vi "S7COMM - Parse Response - Decode Data Item.vi"(8 "error in (no error)":errorcluster, 9 "Variable Type":T1=enum."BIT", 11 "Response Data IN":T2 format="0x%02x") -> (0 "error out":errorcluster, 2 "Read Item - Data":i32[](array[numeric]), 3 "Response Data OUT":T2 format="0x%02x")   [LabVIEW 2014, in "S7NetCom.lvclass"]
doc: "____\nCopyright (c) 2019 Hampel Software Engineering (HSE), released under BSD license. More info can be found on https://dokuwiki.hampel-soft.com/code/hse/s7netcom. Original code published by Marc Christenson, Sisu Devices."
uses:
  S7NetCom.lvclass
  Controls/S7NetCom_HexByteArray.ctl
  Controls/S7NetCom_HexByte.ctl
  Controls/S7_Variable_Type.ctl
  S7COMM - Evaluate Response Item Return Code.vi
  S7COMM - Response Item Return Code-error.vi
panel:
  # "More info on https://dokuwiki.hampel-soft.com/code/hse/s7netcom\n\nCopyright (c) 2019, HAMPEL SOFTWARE ENGINEERING (HSE)\nOriginal code developed by Marc Christenson, Sisu Devices\nAll rights reserved.\n\nRedistribution and use in source and binary forms, with or without\nmodification, are permitted provided that the following conditions are met:\n\n1. Redistributions of source code must retain the above copyright\n   notice, this list of conditions and the following disclaimer.\n\n2. Redistributions in binary form must reproduce the above copyright\n   notice, this list of conditions and the following disclaimer in the\n   documentation and/or other materials provided with the distribution.\n\n3. All advertising materials mentioning features or use of this software\n   must display the following acknowledgement:\n   This product includes software developed by HAMPEL SOFTWARE ENGINEERING.\n\n4. Neither the name of HAMPEL SOFTWARE ENGINEERING nor the\n   names of its contributors may be used to endorse or promote products\n   derived from this software without specific prior written permission.\n\nTHIS SOFTWARE IS PROVIDED BY HAMPEL SOFTWARE ENGINEERING ''AS IS'' AND ANY\nEXPRESS OR IMPLIED WARRANTIES, INCLUDING, BUT NOT LIMITED TO, THE IMPLIED\nWARRANTIES OF MERCHANTABILITY AND FITNESS FOR A PARTICULAR PURPOSE ARE\nDISCLAIMED. IN NO EVENT SHALL HAMPEL SOFTWARE ENGINEERING BE LIABLE FOR ANY\nDIRECT, INDIRECT, INCIDENTAL, SPECIAL, EXEMPLARY, OR CONSEQUENTIAL DAMAGES\n(INCLUDING, BUT NOT LIMITED TO, PROCUREMENT OF SUBSTITUTE GOODS OR SERVICES;\nLOSS OF USE, DATA, OR PROFITS; OR BUSINESS INTERRUPTION) HOWEVER CAUSED AND\nON ANY THEORY OF LIABILITY, WHETHER IN CONTRACT, STRICT LIABILITY, OR TORT\n(INCLUDING NEGLIGENCE OR OTHERWISE) ARISING IN ANY WAY OUT OF THE USE OF THIS\nSOFTWARE, EVEN IF ADVISED OF THE POSSIBILITY OF SUCH DAMAGE."
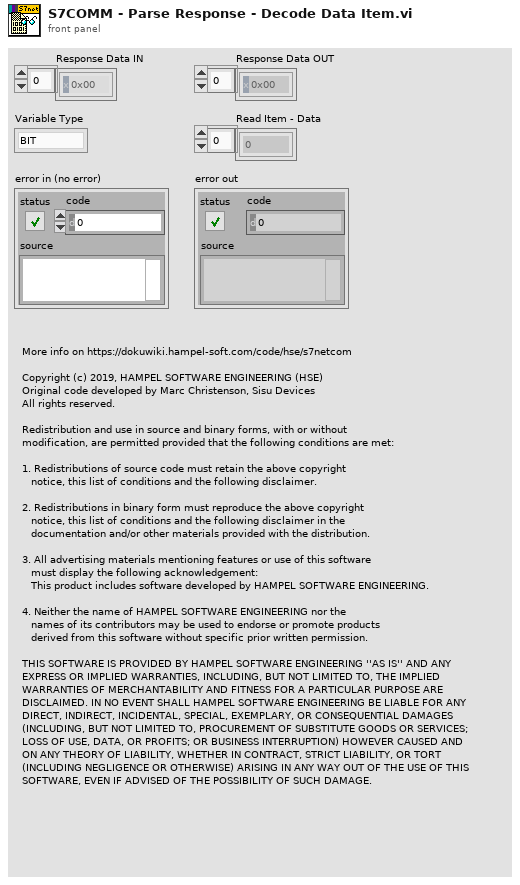
[diagram p1: front panel]
types:
  T1 = typedef "S7NetCom.lvclass/S7_Variable_Type.ctl" = enum8{"---", "BIT", "BYTE", "CHAR", "WORD", "INT", "DWORD", "DINT", "REAL"}
  T2 = typedef "S7NetCom.lvclass/S7NetCom_HexByteArray.ctl" = T3[]
  T3 = typedef "S7NetCom.lvclass/S7NetCom_HexByte.ctl" = u8
  T4 = typedef "S7NetCom.lvclass/S7COMM - Transport Data Types--ring.ctl" = u8
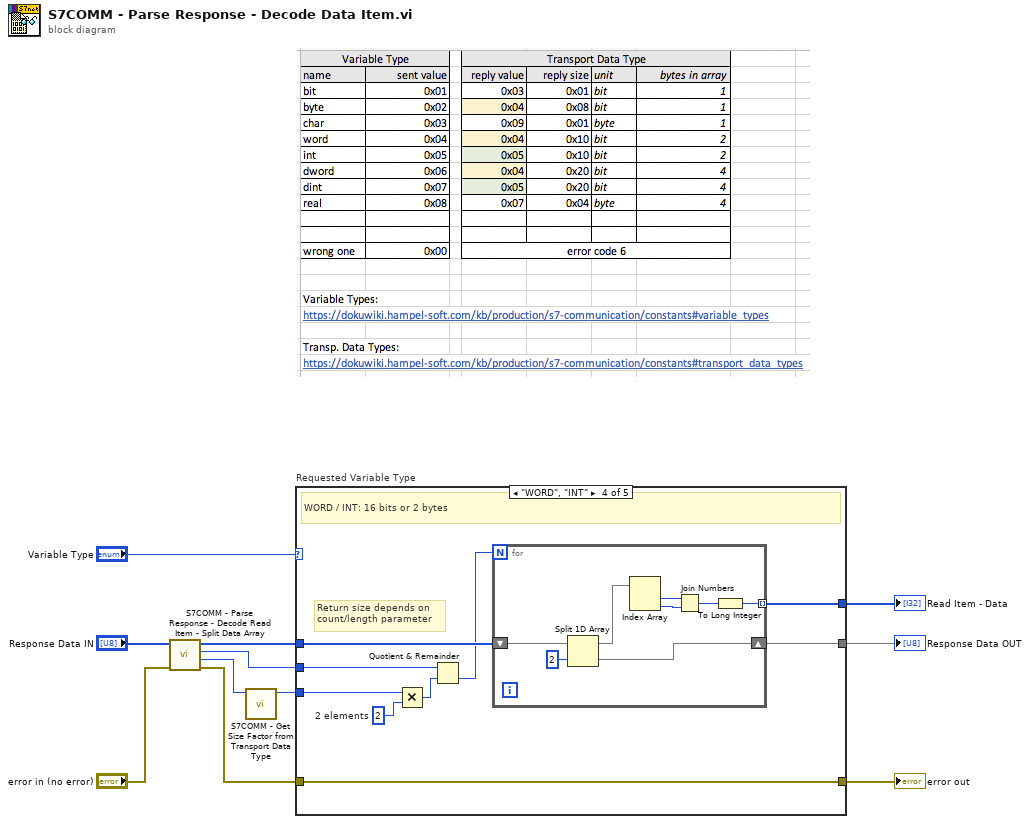
[diagram p0: block diagram]
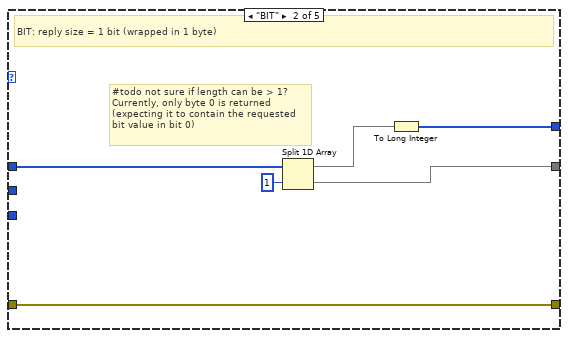
[diagram p3: hidden frame]
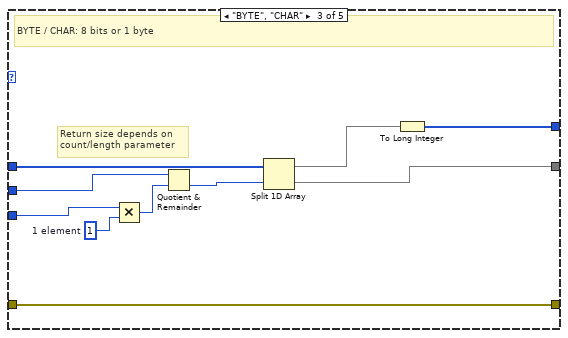
[diagram p4: hidden frame]
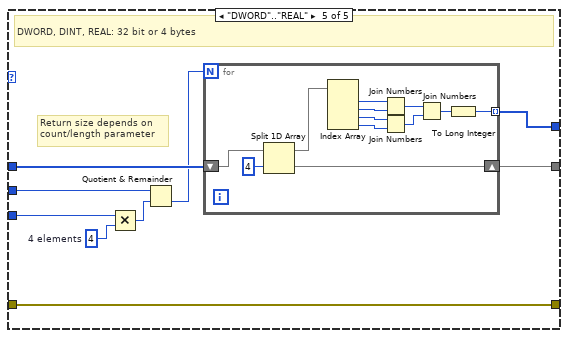
[diagram p5: hidden frame]
diagram:
  n1 = call "S7COMM - Parse Response - Decode Read Item - Split Data Array.vi"("error in (no error)"="error in (no error)", "Response Data IN"="Response Data IN") -> ("error out"=w1:errorcluster, "Transport Data Type"=w6:T4, "Count"=w7:u16, "Rest of Response Data"=w4:T2)  [unwired: 6 in]
  n2 = call "S7COMM - Get Size Factor from Transport Data Type.vi"("Transport Data Type"=w6) -> ("Size Factor"=w8:u16)  [unwired: 10 in]
  n3 = case "Requested Variable Type" shown="\"WORD\", \"INT\"" "Variable Type" {
    tunnel: [_ w19 w24 w35 w53] -> w10
    tunnel: w4 -> [w13 w18 w27 w37 w55]
    tunnel: w7 -> [_ _ w28 w38 w52]
    tunnel: [w13 w17 w26 w36 w54] -> w3
    tunnel: w8 -> [_ _ w22 w31 w49]
    tunnel: [w12 w14 w20 w30 w47] -> w2
    tunnel: w1 -> [w12 w14 w20 w30 w47]
    frame Default {
    }
    frame "BIT" {
      # "#todo not sure if length can be > 1?\nCurrently, only byte 0 is returned \n(expecting it to contain the requested\nbit value in bit 0)"
      # "BIT: reply size = 1 bit (wrapped in 1 byte)"
      n4 = Split 1D Array(array=w18, index=1) -> (first subarray=w16:T2, second subarray=w17:T2)
      n5 = To Long Integer(number=w16) -> (32bit integer=w19:i32[])
    }
    frame "BYTE", "CHAR" {
      w21 = u16 1  # 1 element
      # "Return size depends on \ncount/length parameter"
      # "BYTE / CHAR: 8 bits or 1 byte"
      n6 = Multiply(x=w22, y=w21) -> (x*y=w29:u16)
      n7 = Quotient & Remainder(x=w28, y=w29) -> (floor(x/y)=w23:u16)  [unwired: 1 out]
      n8 = Split 1D Array(array=w27, index=w23) -> (first subarray=w25:T2, second subarray=w26:T2)
      n9 = To Long Integer(number=w25) -> (32bit integer=w24:i32[])
    }
    frame "WORD", "INT" {
      w33 = u16 2  # 2 elements
      # "Return size depends on \ncount/length parameter"
      # "WORD / INT: 16 bits or 2 bytes"
      n10 = Multiply(x=w31, y=w33) -> (x*y=w32:u16)
      n11 = Quotient & Remainder(x=w38, y=w32) -> (floor(x/y)=w34:u16)  [unwired: 1 out]
      n12 = for {
        N: w34 -> [_]
        shift-right: [w45] -> w36
        shift-left: w37 -> [w46]
        tunnel: [w40] -> w35 mode=indexing
        n13 = Split 1D Array(array=w46, index=2) -> (first subarray=w44:T2, second subarray=w45:T2)
        n14 = Index Array(array=w44) -> (element #1=w43:T3, element #2=w42:T3)  [unwired: 2 in]
        n15 = Join Numbers(hi=w43, lo=w42) -> ((hi.lo)=w41:u16)
        n16 = To Long Integer(number=w41) -> (32bit integer=w40:i32)
      }
    }
    frame "DWORD".."REAL" {
      w50 = u16 4  # 4 elements
      # "Return size depends on \ncount/length parameter"
      # "DWORD, DINT, REAL: 32 bit or 4 bytes"
      n17 = Multiply(x=w49, y=w50) -> (x*y=w48:u16)
      n18 = Quotient & Remainder(x=w52, y=w48) -> (floor(x/y)=w51:u16)  [unwired: 1 out]
      n19 = for {
        N: w51 -> [_]
        shift-right: [w66] -> w54
        shift-left: w55 -> [w67]
        tunnel: [w57] -> w53 mode=indexing
        n20 = Split 1D Array(array=w67, index=4) -> (first subarray=w65:T2, second subarray=w66:T2)
        n21 = Index Array(array=w65) -> (element #1=w60:T3, element #2=w59:T3, element #3=w61:T3, element #4=w62:T3)  [unwired: 4 in]
        n22 = Join Numbers(hi=w60, lo=w59) -> ((hi.lo)=w63:u16)
        n23 = Join Numbers(hi=w61, lo=w62) -> ((hi.lo)=w64:u16)
        n24 = Join Numbers(hi=w63, lo=w64) -> ((hi.lo)=w58:u32)
        n25 = To Long Integer(number=w58) -> (32bit integer=w57:i32)
      }
    }
  }
  "Read Item - Data" <- w10
  "Response Data OUT" <- w3
  "error out" <- w2
